vi "testreg_exp4_extracting_name.vi"() -> ()   [LabVIEW 2010]
uses:
  <vilib>/regexp/Match Regular Expression.xnode
panel:
  out "whole match":string
  out "submatch 2":string
  out "submatch 1":string
  in  "input string":string
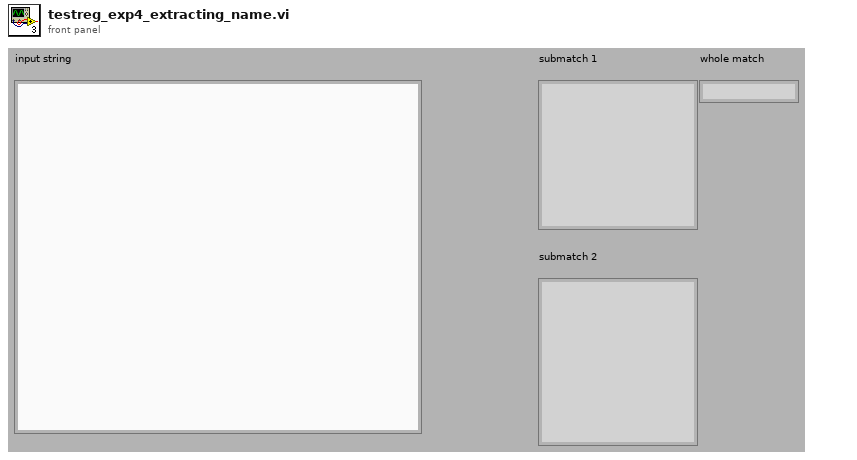
[diagram p1: front panel]
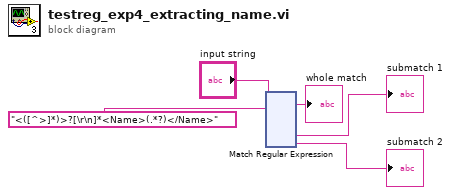
[diagram p0: block diagram]
diagram:
  n1 = xnode "Match Regular Expression"("input string"="input string", "regular expression"="<([^>]*)>?[\r\n]*<Name>(.*?)</Name>") -> ("whole match"=→"whole match":string, "submatch 1"=→"submatch 1":string, "submatch 2"=→"submatch 2":string)  [unwired: 4 in, 4 out]
